vi "RegistroDeDesplazamientos.vi"() -> ()   [LabVIEW 2020]
panel:
  out "x[i-2]":dbl
  out "x[i-1]":dbl
  out "x[i]":dbl
  in  "stop":bool
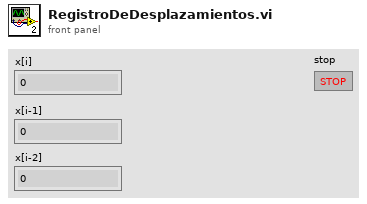
[diagram p1: front panel]
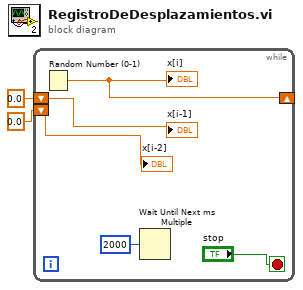
[diagram p0: block diagram]
diagram:
  n1 = while {
    shift-right: [w5] -> _
    shift-left: 0.0 ("number: 0 to 1") -> [w4]
    shift-left: 0.0 ("number: 0 to 1") -> [w3]
    stop <- "stop" stop-if-true
    n2 = Random Number (0-1)() -> (number: 0 to 1=w5:dbl)
    "x[i]" <- w5
    n3 = Wait Until Next ms Multiple(millisecond multiple=u32 2000) -> ()  [unwired: 1 out]
    "x[i-1]" <- w4
    "x[i-2]" <- w3
  }
